vi "Liederberechnung.vi"(10 "to:":dbl, 11 "from:":dbl) -> (0 "ende?":bool, 2 "X:":dbl)   [LabVIEW 2010]
panel:
  in  "zwischenzahl":dbl
  in  "Lieder:":dbl
  # "f+t /2 -1"
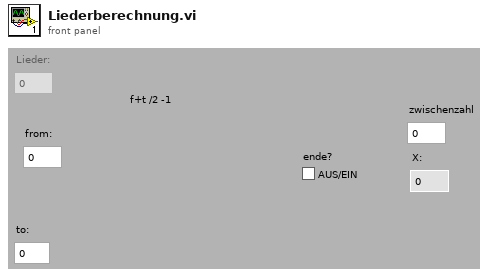
[diagram p1: front panel]
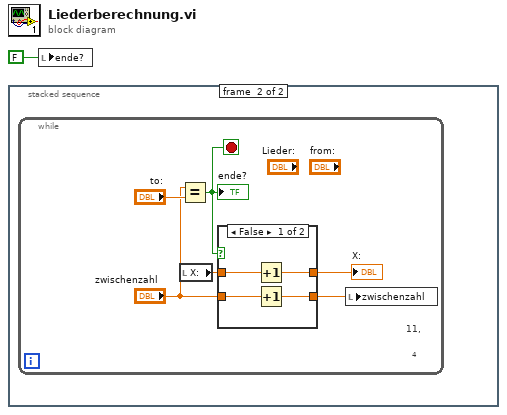
[diagram p0: block diagram]
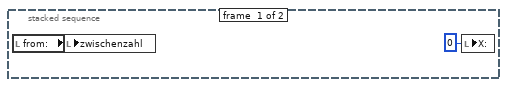
[diagram p2: hidden frame]
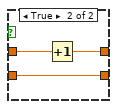
[diagram p3: hidden frame]
diagram:
  n1 = stacked-sequence {
    frame #0 {
      n2 = local read "from:"() -> (w3:dbl)
      n3 = local write "zwischenzahl"(w3) -> ()
      n4 = local write "X:"(0) -> ()
    }
    frame #1 {
      n5 = while {
        stop <- w4 stop-if-true
        # "4"
        # "11,"
        n6 = Equal?(x="zwischenzahl", y="to:") -> (x = y?=w4:bool)
        "ende?" <- w4
        n7 = local read "X:"() -> (w7:dbl)
        n8 = case shown="FALSE" w4 {
          tunnel: "zwischenzahl" -> [w13 w16]
          tunnel: w7 -> [w12 w15]
          tunnel: [w11 w14] -> w6
          tunnel: [w10 w16] -> w5
          frame False {
            n9 = Increment(x=w12) -> (x+1=w11:dbl)
            n10 = Increment(x=w13) -> (x+1=w10:dbl)
          }
          frame True {
            n11 = Increment(x=w15) -> (x+1=w14:dbl)
          }
        }
        "X:" <- w6
        n12 = local write "zwischenzahl"(w5) -> ()
      }
    }
  }
  n13 = local write "ende?"(FALSE) -> ()
